vi "Get Magnet Field.vi"(6 "Axis":T1, 8 "error in (no error)":errorcluster, 11 "Instrument.VRM in":refnum<class "Instrument.OxfordVRM.lvclass">) -> (0 "error out":errorcluster, 1 "Status":variant, 2 "B Field (T)":dbl, 3 "Instrument.VRM out":refnum<class "Instrument.OxfordVRM.lvclass">, 4 "Finished?":bool)   [LabVIEW 2016, in "Instrument.OxfordVRM.lvclass"]
uses:
  Instrument.OxfordVRM.lvclass
  <userlib>/LevyLab/Levylab Instruments/Instrument Types/Cryostat/Typedefs/Magnet Axis--Enum.ctl
  <userlib>/LevyLab/postgreSQL-timescaleDB/Data.PG/API/Read Variable (double).vi
  <userlib>/LevyLab/postgreSQL-timescaleDB/Data.PG/API/Read Variable (string).vi
  <userlib>/LevyLab/postgreSQL-timescaleDB/Data.PG/Data.PGSQL.lvclass
  <userlib>/LevyLab/Levylab Instruments/Instrument Types/Cryostat/Instrument.Cryostat.lvclass
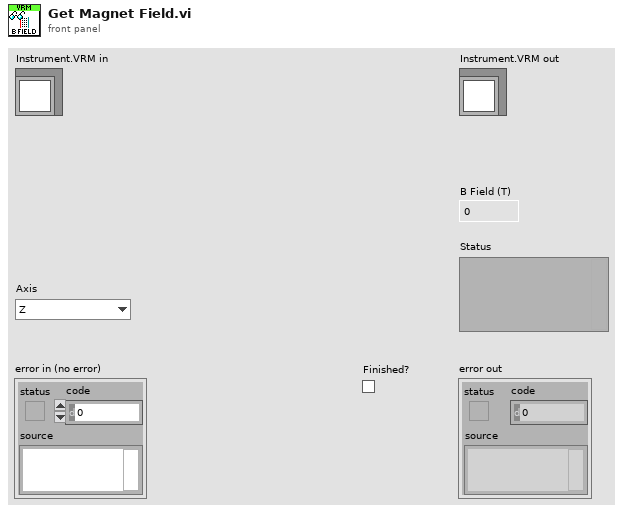
[diagram p1: front panel]
types:
  T1 = typedef "Instrument.Cryostat.lvclass/Magnet Axis--Enum.ctl" = enum16{"Z", "X", "Y"}
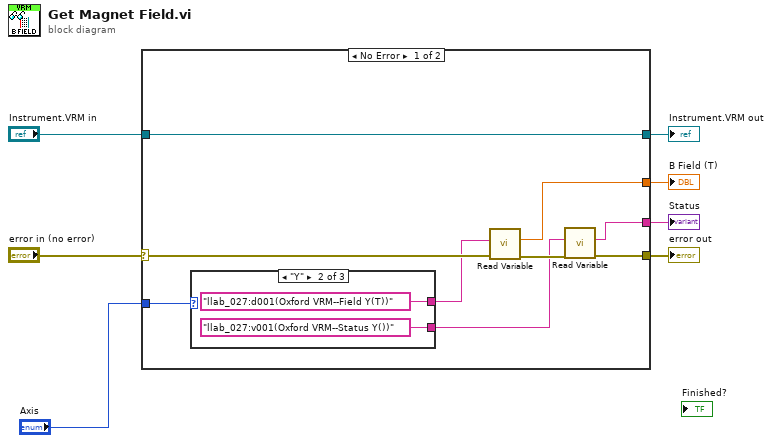
[diagram p0: block diagram]
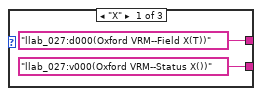
[diagram p2: hidden frame]
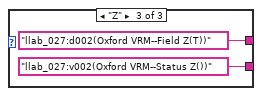
[diagram p3: hidden frame]
diagram:
  n1 = case shown="No Error" "error in (no error)" {
    selector: "error in (no error)" -> [w15 w24]
    tunnel: "Instrument.VRM in" -> [w13 w23]
    tunnel: [w13 w23] -> w6
    tunnel: [w16 _] -> w5
    tunnel: [w14 w24] -> w3
    tunnel: [w12 _] -> w2
    tunnel: "Axis" -> [w10 _]
    frame No Error {
      n2 = case shown="\"Y\"" w10 {
        tunnel: ["llab_027:d000(Oxford VRM--Field X(T))" ("PG path") "llab_027:d001(Oxford VRM--Field Y(T))" ("PG path") "llab_027:d002(Oxford VRM--Field Z(T))" ("PG path")] -> w9
        tunnel: ["llab_027:v000(Oxford VRM--Status X())" ("PG path") "llab_027:v001(Oxford VRM--Status Y())" ("PG path") "llab_027:v002(Oxford VRM--Status Z())" ("PG path")] -> w8
        frame "X" {
        }
        frame "Y" {
        }
        frame "Z" {
        }
      }
      n3 = call-poly <userlib>:"Read Variable.vi"("error in (no error)"=w15, "PG path"=w9) -> ("error out"=w11:errorcluster, "Value"=w16:dbl)  [unwired: 4 in, 4 out]
      n4 = call-poly <userlib>:"Read Variable.vi"("error in (no error)"=w11, "PG path"=w8) -> ("error out"=w14:errorcluster, "Value"=w12:string)  [unwired: 4 in, 4 out]
    }
    frame Error {
    }
  }
  "error out" <- w3
  "Instrument.VRM out" <- w6
  "B Field (T)" <- w5
  "Status" <- w2
